vi "init.vi"(8 "error in (no error)":errorcluster, 11 "Monochromator in":refnum<class "Monochromator.lvclass">) -> (0 "error out":errorcluster, 1 "Emulating":bool, 2 "Initialized":bool, 3 "Monochromator out":refnum<class "Monochromator.lvclass">, 4 "Status":string)   [LabVIEW 2016, in "Monochromator.lvclass"]
uses:
  Monochromator.lvclass
  Monochromator.lvclass/Monochromator.ctl
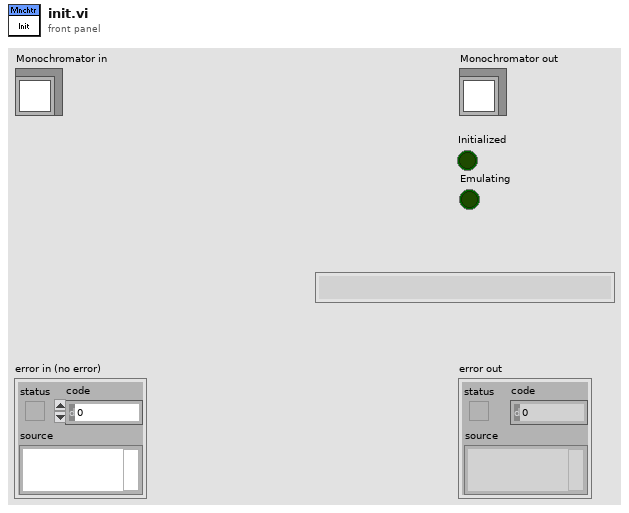
[diagram p1: front panel]
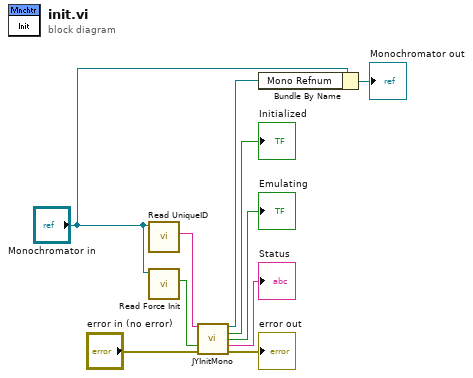
[diagram p0: block diagram]
diagram:
  n1 = call "Read UniqueID.vi"("Monochromator in"="Monochromator in") -> ("UniqueID"=w5:string)  [unwired: 8 in, 2 out]
  n2 = call "Read Force Init.vi"("Monochromator in"="Monochromator in") -> ("Force Init"=w4:bool)  [unwired: 8 in, 2 out]
  n3 = call "JYInitMono.vi"("Unique ID"=w5, "Force Init"=w4, "error in (no error)"="error in (no error)") -> ("Refnum out"=w2:refnum<k7>, "Initialized"=→"Initialized":bool, "Emulating"=→"Emulating":bool, "Status"=→"Status":string, "error out"=→"error out":errorcluster)  [unwired: 8 in]
  n4 = Bundle By Name(cluster="Monochromator in", "Mono Refnum"=w2) -> (→"Monochromator out":refnum<class "Monochromator.lvclass">)
